vi "CLD 16 state machine front panel.vi"() -> ()   [LabVIEW 2009]
doc: "CLD-Übung 16"
uses:
  CLD 16 Control Panel.ctl
  CLD 16 Status Panel.ctl
panel:
  in  "Stopp-Schaltfläche":bool
  out "Produktionsstrecke 2 aktiv":bool
  out "Produktionsstrecke 1 aktiv":bool
  in  "Systemsteuerung - Produktionsstrecke 2":T1
  out "Prozesssteuerung":T2 {"Prozesswert" format="%#.3g"}
  in  "Systemsteuerung - Produktionsstrecke 1":T1
  # "Anzeigepanel"
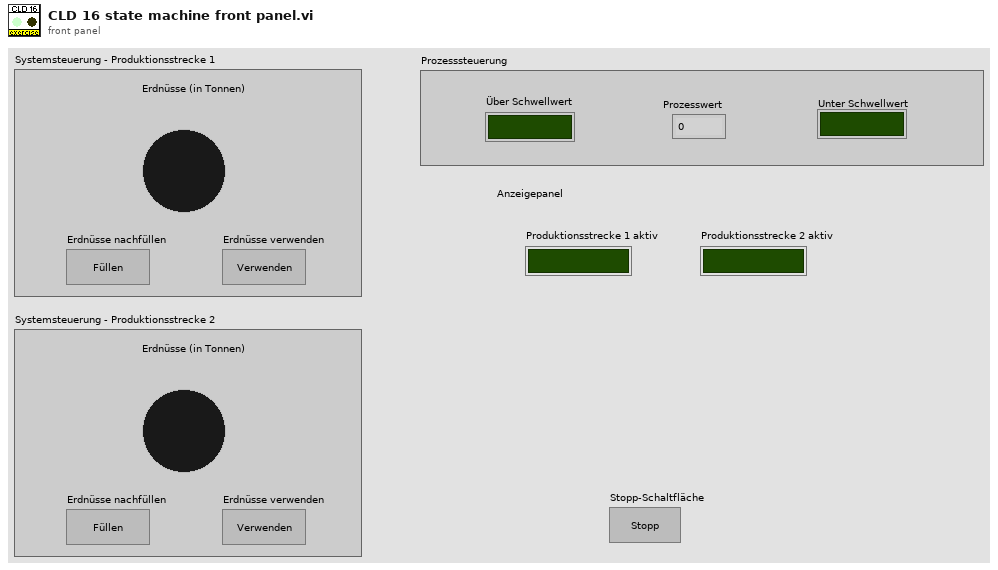
[diagram p1: front panel]
types:
  T1 = typedef "CLD 16 Control Panel.ctl" = cluster{"Erdnüsse (in Tonnen)":i8, "Erdnüsse nachfüllen":bool, "Erdnüsse verwenden":bool}
  T2 = typedef "CLD 16 Status Panel.ctl" = cluster{"Über Schwellwert":bool, "Unter Schwellwert":bool, "Prozesswert":dbl}
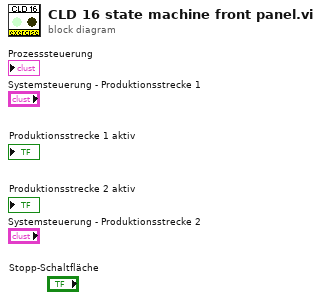
[diagram p0: block diagram]
diagram:
